vi "SGLtoDBL (1 CH).vi"(11 "Waveform in":waveform(sgl)) -> (3 "Waveform out":waveform(dbl))   [LabVIEW 2017, in "McsaAnalysisFunctions.lvlib"]
uses:
  <vilib>/addons/InsightCM/Utilities/Analysis/MCSA/McsaAnalysisFunctions.lvlib
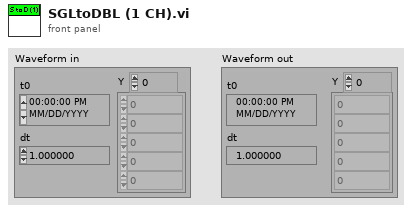
[diagram p1: front panel]
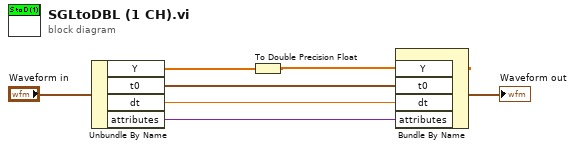
[diagram p0: block diagram]
diagram:
  n1 = Unbundle By Name("Waveform in") -> ("Y"=w2:sgl[], "t0"=w5:timestamp, "dt"=w4:dbl, "attributes"=w3:variant)
  n2 = To Double Precision Float(number=w2) -> (double precision float=w1:dbl[])
  n3 = Bundle By Name("Y"=w1, "t0"=w5, "dt"=w4, "attributes"=w3) -> (→"Waveform out":waveform(dbl))  [unwired: 1 in]
